vi "test_CCDGetDataSize.vi"(7 "Test should pass":bool=TRUE, 8 "error in":errorcluster, 9 "tear down connection":bool=TRUE, 10 "set-up a connection":bool=TRUE, 11 "device selection":enum16{"monochromator", "CCD", "SCD"}(ring)=enum."CCD") -> (0 "error out":errorcluster)   [LabVIEW 2023]
uses:
  Source/Classes/Mono/Monochromator.lvclass
  Source/Classes/CCD/CCD.lvclass
  Source/Classes/SCD/SCD.lvclass
  <vilib>/addons/_JKI Toolkits/Caraya/classes/Assert/Assert Not Error.vi
  <vilib>/addons/_JKI Toolkits/Caraya/classes/Assert/Assert Equal Value and Type_Variant.vi
  Source/Classes/GenericDevice/GenericDevice.lvclass
  <vilib>/addons/_JKI Toolkits/Caraya/classes/Test/Test.lvclass
  <vilib>/addons/_JKI Toolkits/Caraya/classes/Assert/Assert.lvclass
panel:
  # "Connector Pane"
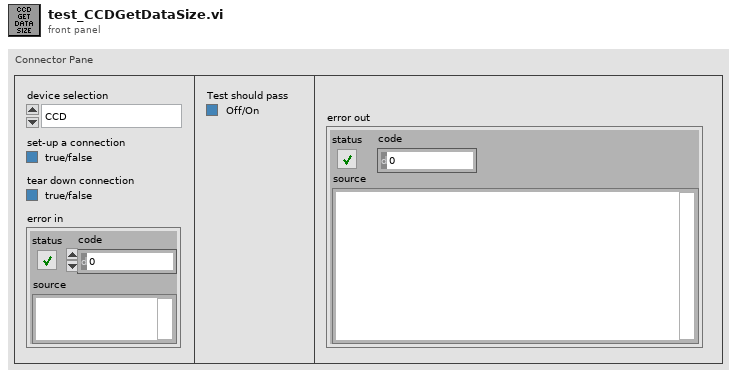
[diagram p1: front panel]
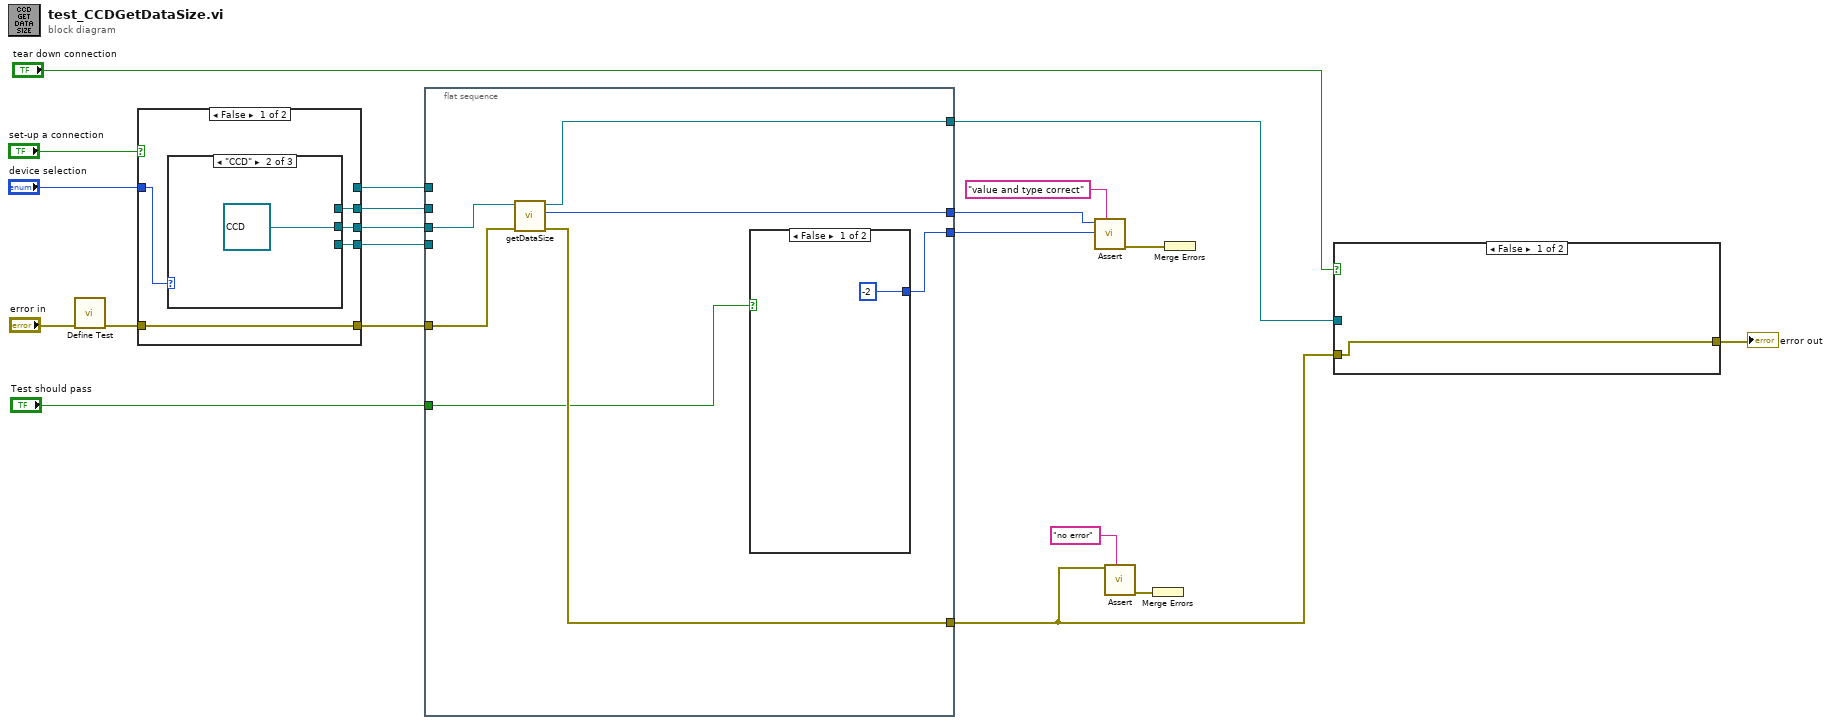
[diagram p0: block diagram]
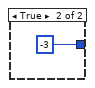
[diagram p2: hidden frame]
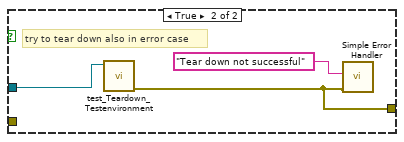
[diagram p3: hidden frame]
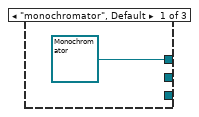
[diagram p4: hidden frame]
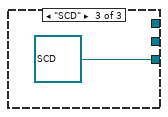
[diagram p5: hidden frame]
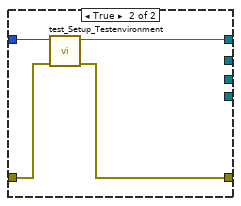
[diagram p6: hidden frame]
diagram:
  n1 = call <vilib>:"Define Test.vi"("error in (no error)"="error in") -> ("error out"=w13:errorcluster)  [unwired: 9 in, 1 out]
  n2 = case shown="False" "set-up a connection" {
    tunnel: w13 -> [w25 w32]
    tunnel: [w25 w31] -> w15
    tunnel: "device selection" -> [w24 w30]
    tunnel: [_ w29] -> w12
    tunnel: [w23 _] -> w11
    tunnel: [w22 _] -> w10
    tunnel: [w21 _] -> w9
    frame False {
      n3 = case shown="\"CCD\"" w24 {
        tunnel: [refnum<class "Monochromator.lvclass"> refnum ("Monochromator.lvclass") _ _] -> w23
        tunnel: [_ refnum<class "CCD.lvclass"> refnum ("CCD in") _] -> w22
        tunnel: [_ _ refnum<class "SCD.lvclass"> refnum ("SCD.lvclass")] -> w21
        frame "monochromator", Default {
        }
        frame "CCD" {
        }
        frame "SCD" {
        }
      }
    }
    frame True {
      n4 = call "test_Setup_Testenvironment.vi"("error in"=w32, "device selection"=w30) -> ("error out"=w31:errorcluster, "GenericDevice.lvclass"=w29:refnum<class "GenericDevice.lvclass">)  [unwired: 7 in, 1 out]
    }
  }
  n5 = flat-sequence {
    tunnel: [w36] -> w17
    tunnel: w15 -> [w39]
    tunnel: w12 -> [_]
    tunnel: w11 -> [_]
    tunnel: w10 -> [w38]
    tunnel: w9 -> [_]
    tunnel: [w35] -> w8
    tunnel: [w37] -> w3
    tunnel: "Test should pass" -> [w34]
    tunnel: [w33] -> w2
    frame #0 {
      n6 = call "getDataSize.vi"("error in (no error)"=w39, "CCD in"=w38) -> ("error out"=w37:errorcluster, "size"=w36:i32, "CCD out"=w33:refnum<class "CCD.lvclass">)  [unwired: 7 in]
      n7 = case shown="False" w34 {
        tunnel: [-2 -3] -> w35
        frame False {
        }
        frame True {
        }
      }
    }
  }
  n8 = call-poly <vilib>:"Assert.vi"("Label"="value and type correct" ("Label (VI Title)"), "Y"=w8, "X"=w17) -> ("error out"=w18:errorcluster)  [unwired: 7 in, 1 out]
  n9 = call-poly <vilib>:"Assert.vi"("Label"="no error" ("Label (VI Title)"), "Not Error?"=w3) -> ("error out"=w5:errorcluster)  [unwired: 8 in, 1 out]
  n10 = Merge Errors(w5) -> ()  [unwired: 1 out]
  n11 = Merge Errors(w18) -> ()  [unwired: 1 out]
  n12 = case shown="False" "tear down connection" {
    tunnel: w2 -> [_ w44]
    tunnel: [w42 w43] -> w1
    tunnel: w3 -> [w42 _]
    frame False {
    }
    frame True {
      # "try to tear down also in error case"
      n13 = call "test_Teardown_Testenvironment.vi"("GenericDevice.lvclass"=w44) -> ("error out"=w43:errorcluster)  [unwired: 9 in, 1 out]
      n14 = call <vilib>:"Simple Error Handler.vi"("error source (\" \")"="Tear down not successful" ("error source (\" \")"), "error in (no error)"=w43) -> ()  [unwired: 3 in, 5 out]
    }
  }
  "error out" <- w1
